vi "RunTimeMenu - Add Channel.vi"(8 "error in (no error)":errorcluster, 11 "Node Ptr":u64 format="%.0x") -> (0 "error out":errorcluster)   [LabVIEW 2016, in "UDP Custom Device System Explorer.lvlib"]
uses:
  UDP Custom Device System Explorer.lvlib
  <vilib>/NI Veristand/Custom Device API/Custom Device Channel.ctl
  <vilib>/NI Veristand/Custom Device API/Custom Device Channel Type.ctl
  <vilib>/NI Veristand/Custom Device API/Custom Device API.lvlib
panel:
  in  "Tag":string
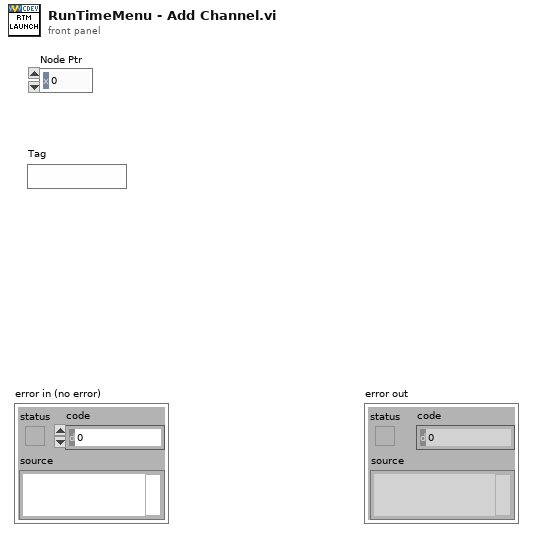
[diagram p1: front panel]
types:
  T1 = typedef "Custom Device API.lvlib/Custom Device Channel Type.ctl" = enum16{"Input", "Output"}
  T2 = typedef "Custom Device API.lvlib/Custom Device Channel.ctl" = cluster{"Type":T1, "Units":string, "Default Value":dbl, "Faultable":bool, "Scalable":bool}
  T3 = typedef "Custom Device API.lvlib/Custom Device Item Ref.ctl" = u64
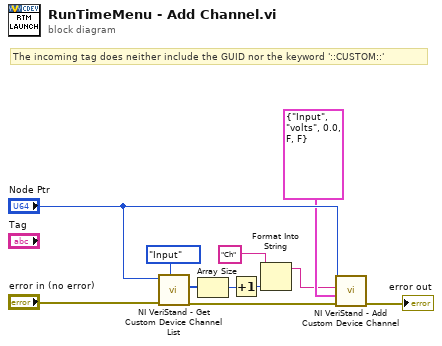
[diagram p0: block diagram]
diagram:
  # "The incoming tag does neither include the GUID nor the keyword '::CUSTOM::'"
  n1 = call <vilib>:"NI VeriStand - Get Custom Device Channel List.vi"("Channel Type"=Custom_Device_Channel_Type."Input", "error in (no error)"="error in (no error)", "Device Ref in"="Node Ptr") -> ("error out"=w8:errorcluster, "Specified Channel Ref List"=w10:T3[])  [unwired: 6 in, 1 out]
  n2 = Array Size(array=w10) -> (size(s)=w2:i32)
  n3 = Increment(x=w2) -> (x+1=w1:i32)
  n4 = Format Into String(initial string="Ch", w1) -> (resulting string=w4:string)  [unwired: 2 in, 1 out]
  n5 = call <vilib>:"NI VeriStand - Add Custom Device Channel.vi"("error in (no error)"=w8, "Channel"=T2 {"Type"=enum."Input", "Units"="volts", "Default Value"=0.0, "Faultable"=FALSE, "Scalable"=FALSE}, "Channel Name"=w4, "Parent Ref in"="Node Ptr") -> ("error out"=→"error out":errorcluster)  [unwired: 4 in, 3 out]
